vi "drawarms.vi"() -> ()   [LabVIEW 2024]
panel:
  in  "x":cluster{"x":dbl, "y":dbl}
  out "end (2D)":cluster{"x":dbl, "y":dbl}
  in  "picture in":picture
  out "end effector":cluster{"X":dbl, "Y":dbl}={"X"=61.080020351084045, "Y"=-1.710100716628343}
  out "2D Picture":picture
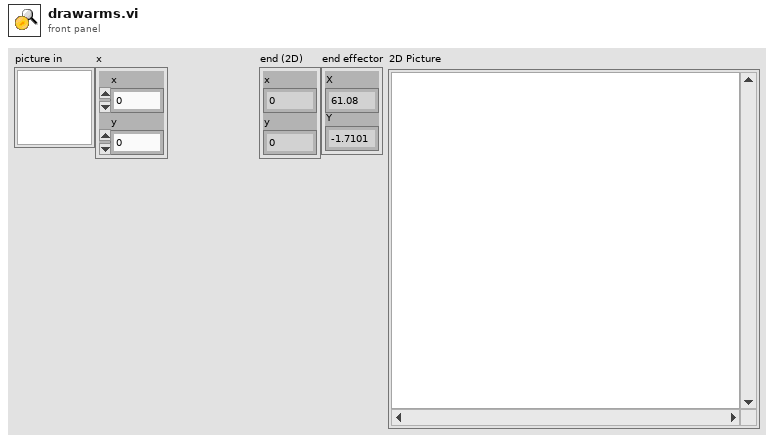
[diagram p1: front panel]
types:
  T1 = cluster{"Width":u16, "Style":enum32{"Solid", "Dash", "Dot", "DashDot", "DashDotDot"}}
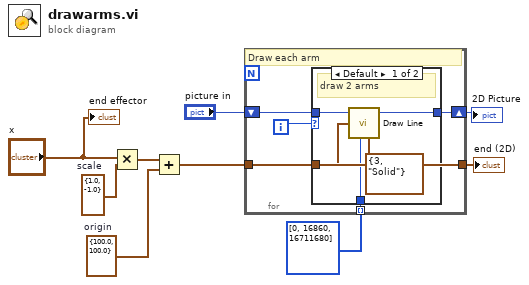
[diagram p0: block diagram]
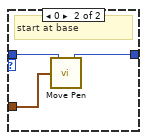
[diagram p2: hidden frame]
diagram:
  w6 = cluster{"x":dbl, "y":dbl} {"x"=1.0, "y"=-1.0}  # scale
  w5 = cluster{"x":dbl, "y":dbl} {"x"=100.0, "y"=100.0}  # origin
  n1 = Multiply(x="x", y=w6) -> (x*y=w4:cluster{"x":dbl, "y":dbl})
  n2 = Add(x=w4, y=w5) -> (x+y=w3:cluster{"x":dbl, "y":dbl})
  n3 = for {
    shift-right: [w12] -> w9
    shift-left: "picture in" -> [w13]
    tunnel: u32[] [0, 16860, 16711680] -> [w11] mode=indexing
    tunnel: w3 -> [w10]
    tunnel: [w10] -> w2
    i -> [w14]
    # "Draw each arm"
    n4 = case shown="Default" w14 {
      tunnel: w13 -> [w19 w22]
      tunnel: [w18 w21] -> w12
      tunnel: w10 -> [w17 w20]
      tunnel: w11 -> [w16 _]
      frame Default {
        # "draw 2 arms"
        n5 = call <vilib>:"Draw Line.vi"("picture"=w19, "end point"=w17, "color(black)"=w16, "pen"=T1 {"Width"=3, "Style"=enum."Solid"}) -> ("new picture"=w18:picture)  [unwired: 5 in]
      }
      frame 0 {
        # "start at base"
        n6 = call <vilib>:"Move Pen.vi"("new position"=w20, "picture"=w22) -> ("new picture"=w21:picture)  [unwired: 3 in]
      }
    }
  }
  "2D Picture" <- w9
  "end (2D)" <- w2
  "end effector" <- "x"
